vi "Set Arm or Winch Global.vi"(1 "error in":errorcluster, 2 "Button B":bool, 3 "Button A":bool) -> (0 "error out":errorcluster)   [LabVIEW 2017]
uses:
  Global Arm Variables.vi
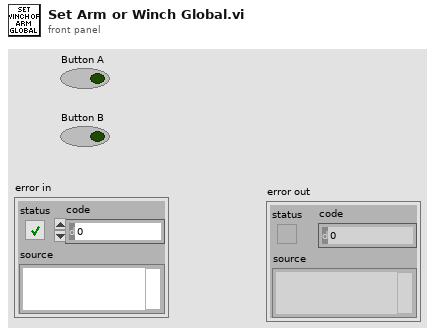
[diagram p1: front panel]
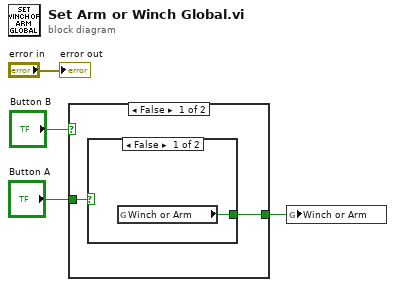
[diagram p0: block diagram]
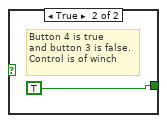
[diagram p2: hidden frame]
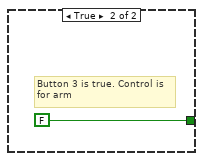
[diagram p3: hidden frame]
diagram:
  n1 = case shown="False" "Button B" {
    tunnel: [w6 FALSE] -> w2
    tunnel: "Button A" -> [w5 _]
    frame False {
      n2 = case shown="False" w5 {
        tunnel: [w7 TRUE] -> w6
        frame False {
          n3 = global read "Global Arm Variables.vi" "Winch or Arm"() -> (w7:bool)
        }
        frame True {
          # "Button 4 is true\nand button 3 is false.\nControl is of winch"
        }
      }
    }
    frame True {
      # "Button 3 is true. Control is\nfor arm"
    }
  }
  n4 = global write "Global Arm Variables.vi" "Winch or Arm"(w2) -> ()
  "error out" <- "error in"
